vi "RSZVB Load And Interchange Balanced Port Circuit Model Data.vi"(5 "Parameter (Port 1)":i32(ring) items=["Port 1", "Port 2"], 6 "File Name (\"\")":string, 7 "Logical Port Number (1)":i32=1, 8 "error in (no error)":errorcluster {"code" format="%.0x"}, 9 "Function Type (Deembedding)":i32(ring) items=["Deembedding", "Embedding"], 10 "Channel (1)":i32=1, 11 "VISA session":refnum<visa-resource-name>) -> (0 "error out":errorcluster {"code" format="%.0x"}, 3 "dup VISA session":refnum<visa-resource-name>)   [LabVIEW 2011]
doc: "This VI loads data from a specified Touchstone file defining the characteristics of the current embedded/deembedded balanced port circuit model. A balanced port circuit model involving file import must be selected before using this VI. \n\nRemote-control command(s):\nMMEMory:LOAD:VNETworks<Ch>:BALanced:EMBedding<Log_pt> '<file_name>', PMAin | PSECondary \nMMEMory:LOAD:VNETworks<Ch>:BALanced:DEEMbedding<Log_pt> '<file_name>', PMAin | PSECondary"
uses:
  _utility/RSZVB Global Data.vi
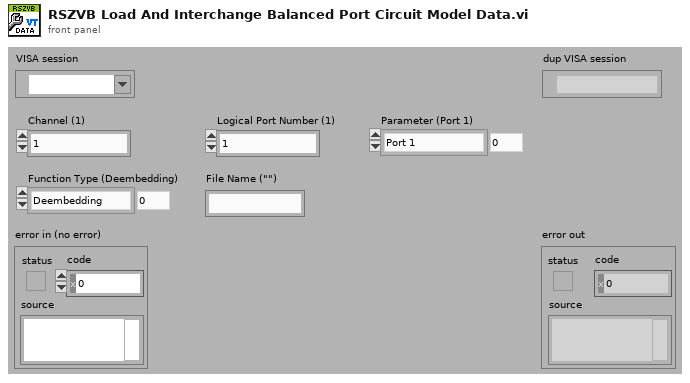
[diagram p1: front panel]
types:
  T1 = cluster{"Error Checking (T: On)":bool, "Installed Options":string[], "Data Valid?":bool, "Ports":i32, "Model":string[], "Option Checking (T: On)":bool}[]
  T2 = cluster{"Error Checking (T: On)":bool, "Installed Options":string[], "Data Valid?":bool, "Ports":i32, "Model":string[], "Option Checking (T: On)":bool}
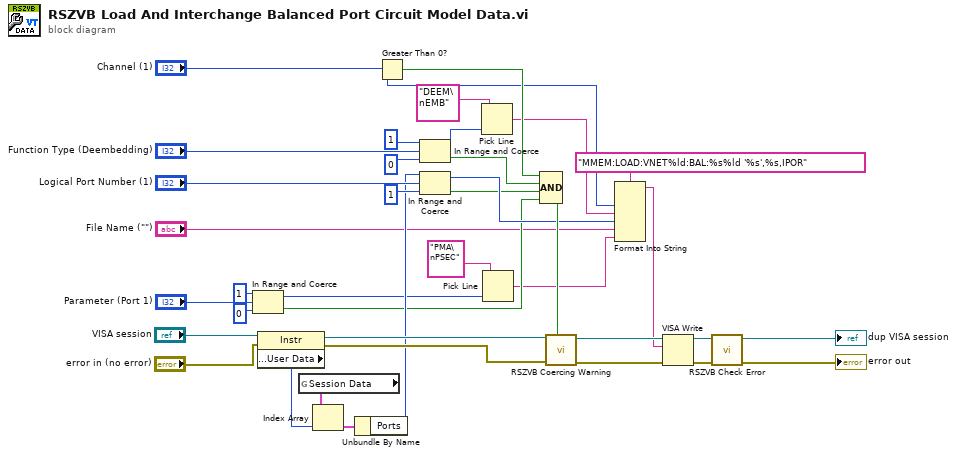
[diagram p0: block diagram]
diagram:
  n1 = In Range and Coerce(upper limit=1, x="Parameter (Port 1)", lower limit=0) -> (coerced(x)=w9:i32, In Range?=w7:bool)
  n2 = property class="Instr"(reference="VISA session", error in="error in (no error)") -> (reference out=w28:refnum<visa-resource-name>, error out=w29:errorcluster, "General Settings:User Data"=w32:u32)
  n3 = global read "RSZVB Global Data.vi" "Session Data"() -> (w31:T1)
  n4 = Index Array(array=w31, index=w32) -> (element=w30:T2)
  n5 = Unbundle By Name(w30) -> ("Ports"=w11:i32)
  n6 = Greater Than 0?(x="Channel (1)") -> (x > 0?=w25:bool)
  n7 = In Range and Coerce(upper limit=1 ("lower limit"), x="Function Type (Deembedding)", lower limit=0) -> (coerced(x)=w19:i32, In Range?=w22:bool)
  n8 = In Range and Coerce(upper limit=w11, x="Logical Port Number (1)", lower limit=1) -> (coerced(x)=w21:i32, In Range?=w17:bool)
  n9 = Pick Line(multi-line string="DEEM\nEMB", line index=w19) -> (output string=w18:string)  [unwired: 1 in]
  n10 = Pick Line(multi-line string="PMA\nPSEC", line index=w9) -> (output string=w2:string)  [unwired: 1 in]
  n11 = Compound Arithmetic op=AND(w25, w22, w17, w7) -> (w24:bool)
  n12 = call "RSZVB Coercing Warning.vi"("In Range?"=w24, "error in (no error)"=w29, "VISA session"=w28) -> ("error out"=w37:errorcluster, "dup VISA session"=w38:refnum<visa-resource-name>)  [unwired: 7 in]
  n13 = Format Into String(format string="MMEM:LOAD:VNET%ld:BAL:%s%ld '%s',%s,IPOR", "Channel (1)", w18, w21, "File Name (\"\")", w2) -> (resulting string=w33:string)  [unwired: 2 in, 1 out]
  n14 = VISA Write(VISA resource name=w38, write buffer=w33, error in (no error)=w37) -> (VISA resource name out=w35:refnum<visa-resource-name>, error out=w36:errorcluster)  [unwired: 1 out]
  n15 = call "RSZVB Check Error.vi"("error in (no error)"=w36, "VISA session"=w35) -> ("error out"=→"error out":errorcluster, "dup VISA session"=→"dup VISA session":refnum<visa-resource-name>)  [unwired: 8 in]
